vi "Configure DC Current.vi"(6 "NPLC":u16(ring)=1 items=["0.00005", "1", "12", "15"], 7 "Aperture Seconds":dbl, 8 "error in (no error)":errorcluster, 9 "Manual Range":dbl=3.0, 10 "Auto Range? (T: Auto)":bool, 11 "VISA resource name":refnum<visa-resource-name>) -> (0 "error out":errorcluster, 3 "VISA resource name out":refnum<visa-resource-name>)   [LabVIEW 2016, in "Keithley DMM7510.lvlib"]
doc: "This VI configures the DC Current measurement and the related parameters."
uses:
  Keithley DMM7510.lvlib
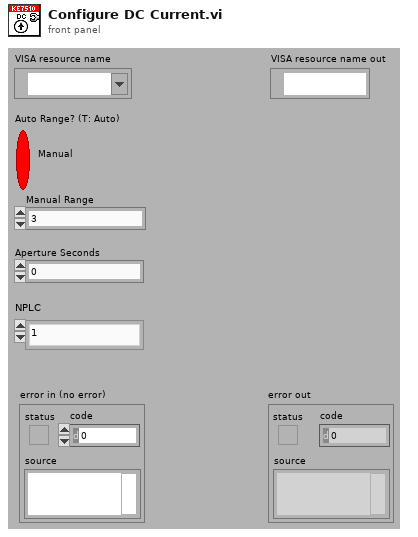
[diagram p1: front panel]
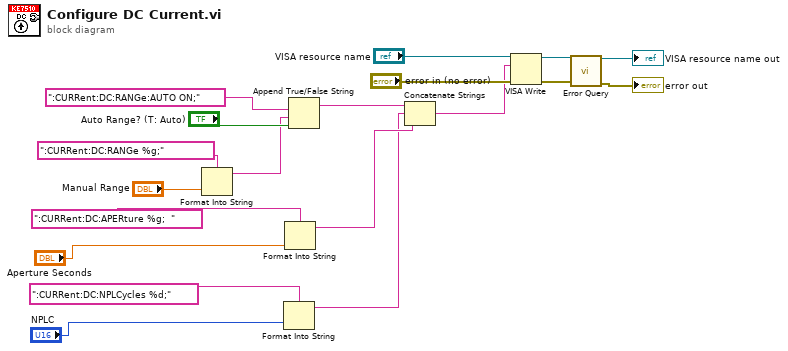
[diagram p0: block diagram]
diagram:
  n1 = Format Into String(format string=":CURRent:DC:RANGe %g;", "Manual Range") -> (resulting string=w13:string)  [unwired: 2 in, 1 out]
  n2 = Format Into String(format string=":CURRent:DC:NPLCycles %d;", "NPLC") -> (resulting string=w1:string)  [unwired: 2 in, 1 out]
  n3 = Format Into String(format string=":CURRent:DC:APERture %g;  ", "Aperture Seconds") -> (resulting string=w2:string)  [unwired: 2 in, 1 out]
  n4 = Append True/False String(1:"Auto Range? (T: Auto)", 2:w13, 3:":CURRent:DC:RANGe:AUTO ON;") -> (0:w10:string)  [unwired: 1 in]
  n5 = Concatenate Strings(w10, w1, w2) -> (w9:string)
  n6 = VISA Write(VISA resource name="VISA resource name", write buffer=w9, error in (no error)="error in (no error)") -> (VISA resource name out=w8:refnum<visa-resource-name>, error out=w7:errorcluster)  [unwired: 1 out]
  n7 = call "Error Query.vi"("error in (no error)"=w7, "VISA resource name"=w8) -> ("error out"=→"error out":errorcluster, "VISA resource name out"=→"VISA resource name out":refnum<visa-resource-name>)  [unwired: 6 in, 2 out]
